vi "initialise.vi"(8 "error in (no error)":errorcluster, 11 "Refnum in":refnum<k34>) -> (0 "error out":errorcluster, 1 "Numeric Control":i32, 2 "Resistance @ Room Temperature (ohms)":dbl, 3 "Heating up":bool, 5 "Room Temperature (K)":dbl)   [LabVIEW 2013]
uses:
  Controls/FGV Function.ctl
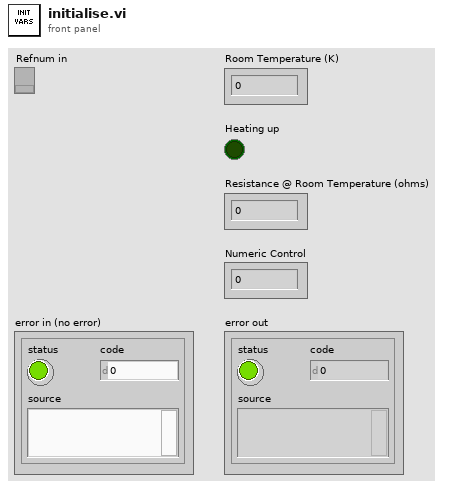
[diagram p1: front panel]
types:
  T1 = typedef "FGV Function.ctl" = enum16{"Initiate", "Read", "Set On", "Set Off"}
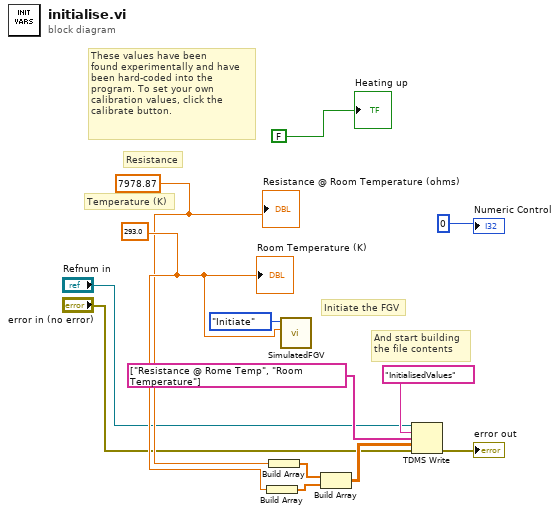
[diagram p0: block diagram]
diagram:
  w9 = 293.0
  w8 = 7978.87
  # "And start building\nthe file contents"
  # "Initiate the FGV"
  # "Temperature (K)"
  # "Resistance"
  # "These values have been\nfound experimentally and have\nbeen hard-coded into the \nprogram. To set your own \ncalibration values, click the\ncalibrate button."
  n1 = Build Array(w9) -> (w10:dbl[])
  n2 = Build Array(w8) -> (w11:dbl[])
  n3 = call "SimulatedFGV.vi"("Starting Temperature"=w9, "FGV Function"=FGV_Function."Initiate") -> ()  [unwired: 9 in, 1 out]
  n4 = Build Array(w11, w10) -> (w12:dbl[][])
  n5 = TDMS Write(0:"Refnum in", 5:"InitialisedValues", 7:string[] ["Resistance @ Rome Temp", "Room Temperature"], 9:w12, 11:"error in (no error)") -> (15:→"error out":errorcluster)  [unwired: 1 in, 3 out]
  "Resistance @ Room Temperature (ohms)" <- w8
  "Room Temperature (K)" <- w9
  "Heating up" <- FALSE ("Voltage")
  "Numeric Control" <- 0
